vi "Dictionary Test - 002.vi"(8 "error in (no error)":errorcluster) -> (0 "error out":errorcluster, 2 "pass":bool)   [LabVIEW 2009]
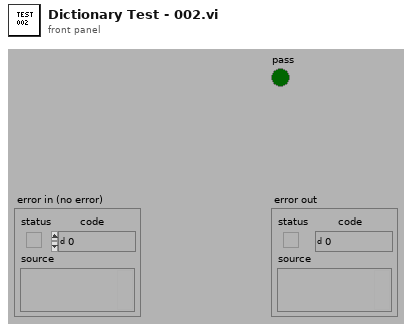
[diagram p1: front panel]
types:
  T1 = typedef "Dictionary Object RefNum.ctl" = refnum<k1>
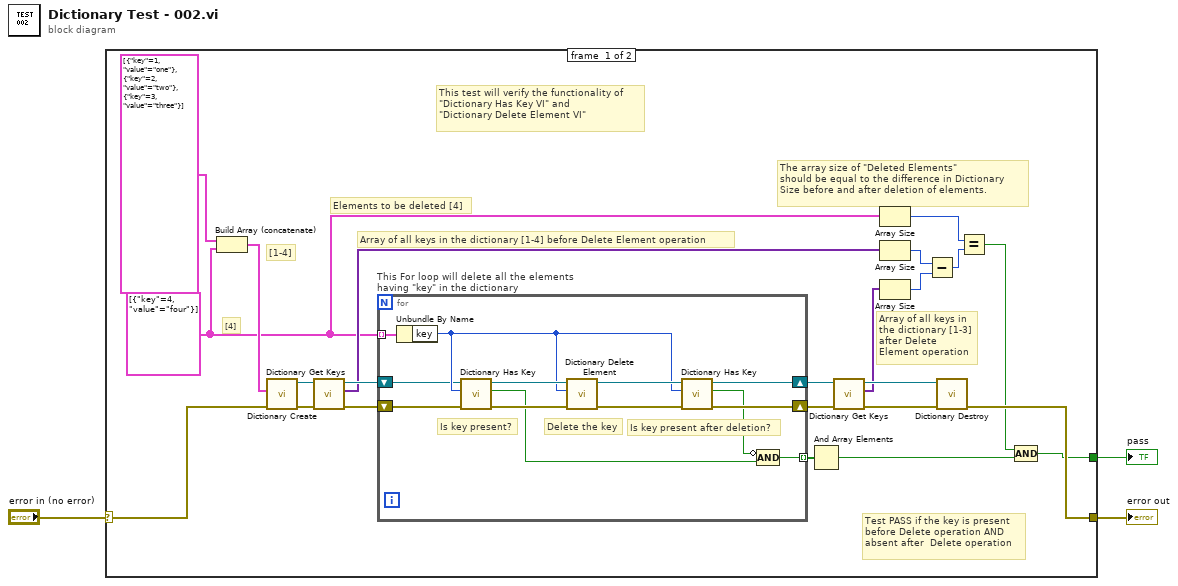
[diagram p0: block diagram]
diagram:
  n1 = case shown="No Error" "error in (no error)" {
    selector: "error in (no error)" -> [w26 w40]
    tunnel: [w25 w40] -> w1
    tunnel: [w8 _] -> w3
    frame #0 {
      w6 = cluster{"key":i32, "value":string}[] [{"key"=4, "value"="four"}]
      # "Array of all keys in the dictionary [1-3]\nafter Delete Element operation"
      # "Array of all keys in the dictionary [1-4] before Delete Element operation"
      # "Elements to be deleted [4]"
      # "The array size of \"Deleted Elements\"\nshould be equal to the difference in Dictionary \nSize before and after deletion of elements."
      # "This test will verify the functionality of \n\"Dictionary Has Key VI\" and \n\"Dictionary Delete Element VI\""
      # "Test PASS if the key is present \nbefore Delete operation AND \nabsent after  Delete operation"
      # "[4]"
      # "[1-4]"
      n2 = Build Array (concatenate)(cluster{"key":i32, "value":string}[] [{"key"=1, "value"="one"}, {"key"=2, "value"="two"}, {"key"=3, "value"="three"}] ("dictionary with updates"), w6) -> (w23:cluster{"key":i32, "value":string}[])
      n3 = call "Dictionary Create.vi"("error in (no error)"=w26, "initial dictionary (empty)"=w23) -> ("error out"=w21:errorcluster, "dictionary out"=w20:T1)  [unwired: 8 in]
      n4 = call "Dictionary Get Keys.vi"("error in (no error)"=w21, "dictionary"=w20) -> ("error out"=w22:errorcluster, "keys"=w18:variant[], "dictionary out"=w19:T1)  [unwired: 7 in]
      n5 = for "This For loop will delete all the elements having \"key\" in the dictionary" {
        tunnel: w6 -> [w34] mode=indexing
        shift-right: [w33] -> w17
        shift-left: w22 -> [w32]
        shift-right: [w31] -> w16
        shift-left: w19 -> [w30]
        tunnel: [w27] -> w10 mode=indexing
        # "Is key present after deletion?"
        # "Delete the key"
        # "Is key present?"
        n6 = Unbundle By Name(w34) -> ("key"=w35:i32)
        n7 = call "Dictionary Has Key.vi"("error in (no error)"=w32, "key"=w35, "dictionary"=w30) -> ("error out"=w36:errorcluster, "Has Key?"=w28:bool, "dictionary out"=w37:T1)  [unwired: 6 in]
        n8 = call "Dictionary Delete Element.vi"("error in (no error)"=w36, "key"=w35, "dictionary"=w37) -> ("error out"=w39:errorcluster, "dictionary out"=w38:T1)  [unwired: 7 in]
        n9 = call "Dictionary Has Key.vi"("error in (no error)"=w39, "key"=w35, "dictionary"=w38) -> ("error out"=w33:errorcluster, "Has Key?"=w29:bool, "dictionary out"=w31:T1)  [unwired: 6 in]
        n10 = Compound Arithmetic op=AND(invert w29, w28) -> (w27:bool)
      }
      n11 = And Array Elements(Boolean array=w10) -> (logical AND=w9:bool)
      n12 = call "Dictionary Get Keys.vi"("error in (no error)"=w17, "dictionary"=w16) -> ("error out"=w14:errorcluster, "keys"=w13:variant[], "dictionary out"=w15:T1)  [unwired: 7 in]
      n13 = Array Size(array=w6) -> (size(s)=w5:i32)
      n14 = Array Size(array=w18) -> (size(s)=w12:i32)
      n15 = Array Size(array=w13) -> (size(s)=w11:i32)
      n16 = Subtract(x=w12, y=w11) -> (x-y=w4:i32)
      n17 = call "Dictionary Destroy.vi"("error in (no error)"=w14, "dictionary"=w15) -> ("error out"=w25:errorcluster)  [unwired: 9 in]
      n18 = Equal?(x=w5, y=w4) -> (x = y?=w7:bool)
      n19 = Compound Arithmetic op=AND(w7, w9) -> (w8:bool)
    }
    frame #1 {
    }
  }
  "pass" <- w3
  "error out" <- w1
